vi "Reset.vi"(8 "error in (no error)":errorcluster, 11 "AbstractCollector1D in":refnum<class "AbstractCollector1D.lvclass">) -> (0 "error out":errorcluster, 3 "AbstractCollector1D out":refnum<class "AbstractCollector1D.lvclass">)   [LabVIEW 2014, in "AbstractCollector1D.lvclass"]
uses:
  AbstractCollector1D.lvclass
  Model/Data/Data1D/Data1D.lvclass
  AbstractCollector/AbstractCollector.lvclass
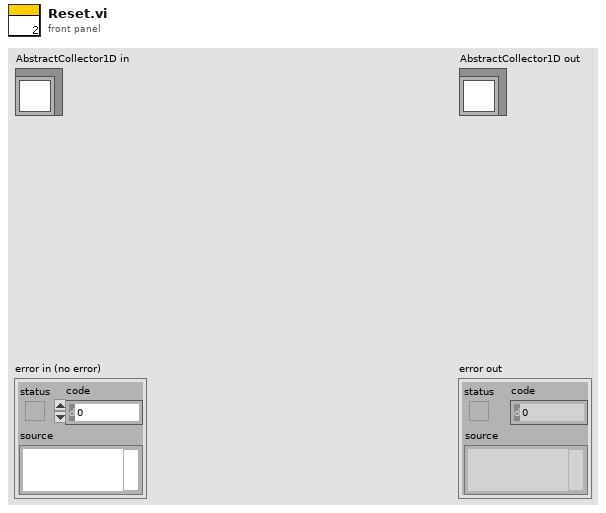
[diagram p1: front panel]
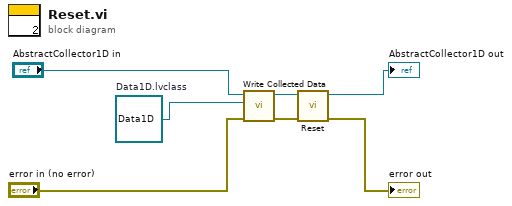
[diagram p0: block diagram]
diagram:
  w1 = refnum<class "Data1D.lvclass"> refnum  # Data1D.lvclass
  n1 = call-dynamic "Write Collected Data.vi"("error in (no error)"="error in (no error)", "Collected Data"=w1, "AbstractCollector in"="AbstractCollector1D in") -> ("error out"=w4:errorcluster, "AbstractCollector out"=w5:refnum<class "AbstractCollector1D.lvclass">)  [unwired: 7 in]
  n2 = call-parent "Reset.vi"("error in (no error)"=w4, "AbstractCollector in"=w5) -> ("error out"=→"error out":errorcluster, "AbstractCollector out"=→"AbstractCollector1D out":refnum<class "AbstractCollector1D.lvclass">)  [unwired: 8 in]
